vi "XYZStage-Initialisation (ver 2).vi"(8 "Error In":errorcluster, 10 "Stage Comms":T1={"CommsProtocol.lvclass"=refnum, "CommsProtocol.lvclass 2"=refnum, "CommsProtocol.lvclass 3"=refnum, "XYZ Control Config"=enum."XYZ", "Translation Stage Description"=""}, 11 "XYZ Stage Control.lvclass":refnum<class "XYZ Stage Control.lvclass">) -> (0 "Error Out":errorcluster, 3 "XYZ Stage Control out":refnum<class "XYZ Stage Control.lvclass">)   [LabVIEW 2020]
uses:
  Typedefs/Comms settings-rs232.ctl
  XYZ Stage Control/XYZ Stage Control.lvclass
  typedefs/TranslationStageControlInfo.ctl
  Generic Comms/CommsProtocol/CommsProtocol.lvclass
  typedefs/XYZControlConfig.ctl
  Globals/gl_XYZStage globals.vi
  <instrlib>/Olympus IX BX Series/Olympus IX BX Series.lvlib
  <vilib>/Instr/_visa.llb/VISA Configure Serial Port (Instr).vi
panel:
  in  "Connection Z":T3={"baud rate"=9600, "data bits"=8, "parity"=0, "stop bits"=10, "flow control"=0} {"flow control" items=["None"=0, "XON/XOFF"=1, "RTS/CTS"=2, "DTR/DSR"=4]; "stop bits" items=["1.0"=10, "1.5"=15, "2.0"=20]; "parity" items=["None", "Odd", "Even", "Mark", "Space"]; "data bits" min=5 max=8 step=1}
  out "VISA resource name out Z":refnum<visa-resource-name>
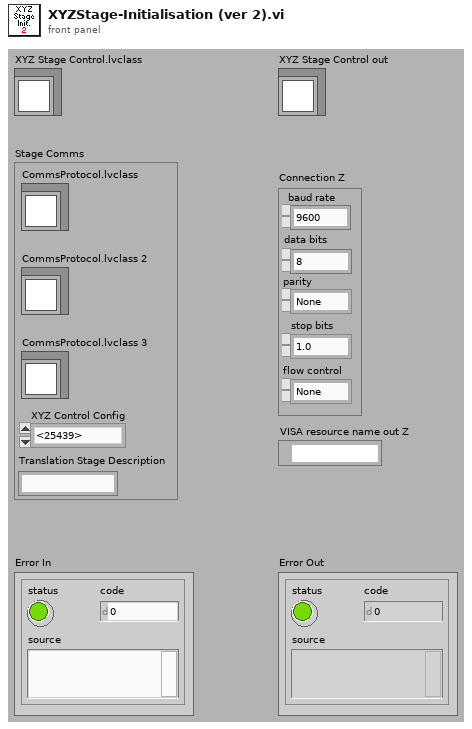
[diagram p1: front panel]
types:
  T1 = typedef "TranslationStageControlInfo.ctl" = cluster{"CommsProtocol.lvclass":refnum<class "CommsProtocol.lvclass">, "CommsProtocol.lvclass 2":refnum<class "CommsProtocol.lvclass">, "CommsProtocol.lvclass 3":refnum<class "CommsProtocol.lvclass">, "XYZ Control Config":T2, "Translation Stage Description":string}
  T2 = typedef "XYZControlConfig.ctl" = enum16{"None", "XYZ", "XY-Z", "X-Y-Z", "Z"}
  T3 = typedef "Comms settings-rs232.ctl" = cluster{"baud rate":u32, "data bits":u16, "parity":u16, "stop bits":u16, "flow control":u16}
  T4 = cluster{"Baud Rate (19200)":u32, "Flow Control (2: RTS/CTS)":u16, "Parity (2: Even)":u16, "Data Bits (8)":u16, "Stop Bits (20: 2.0)":u16}
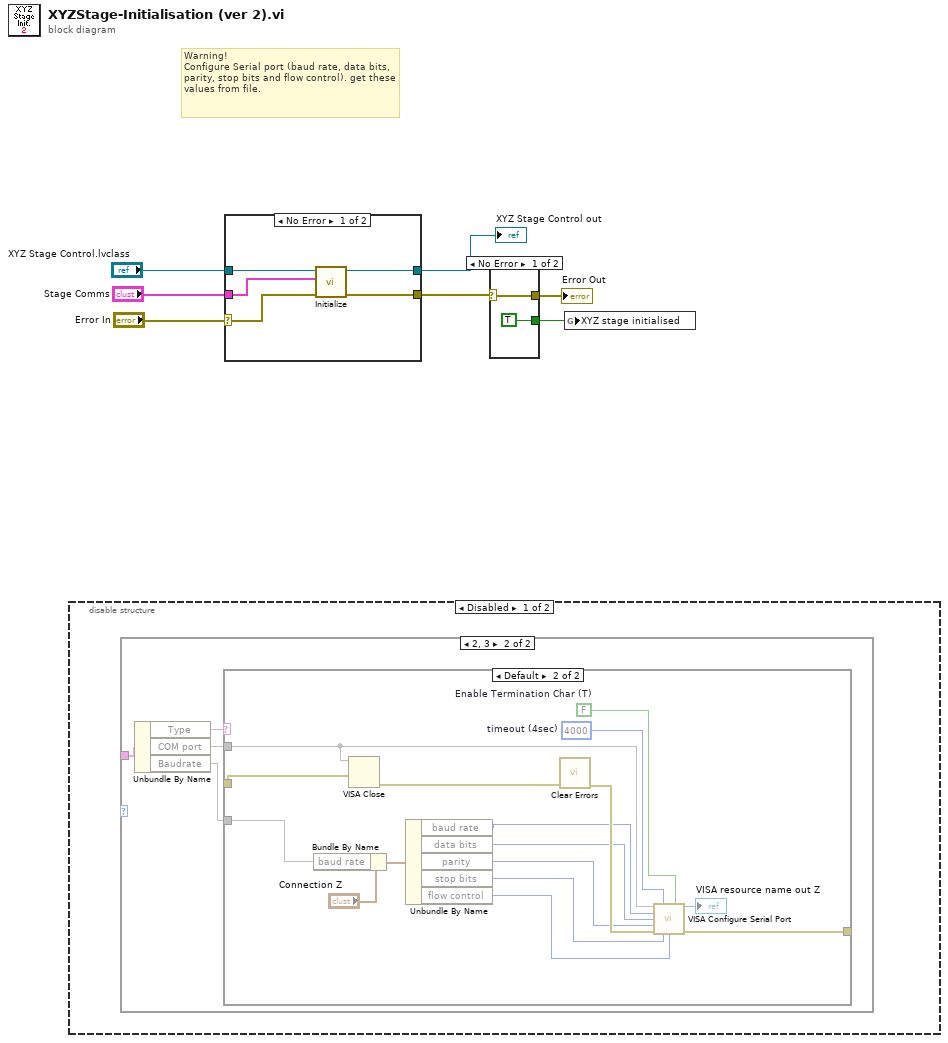
[diagram p0: block diagram]
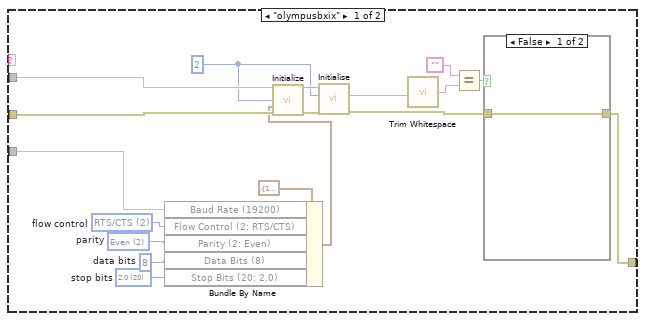
[diagram p3: hidden frame]
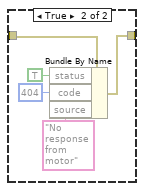
[diagram p4: hidden frame]
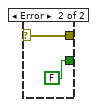
[diagram p6: hidden frame]
diagram:
  # "Warning!\nConfigure Serial port (baud rate, data bits, parity, stop bits and flow control). get these values from file."
  n1 = disable-structure shown="Disabled" {
    frame Disabled {
      n2 = case shown="2, 3" {
        selector: _ -> [_ _]
        tunnel: _ -> [_ w10]
        frame 0, Default {
        }
        frame 2, 3 {
          n3 = Unbundle By Name(w10) -> ("Type"=w8, "COM port"=w12, "Baudrate"=w11)
          n4 = case shown="Default" w8 {
            tunnel: w12 -> [w25 w49]
            tunnel: w11 -> [w26 w45]
            tunnel: [w28 w40] -> w9
            tunnel: [w20 w39] -> _
            frame "olympusbxix" {
              w18 = u16 8  # data bits
              w17 = u16 2 items=["None", "Odd", "Even", "Mark", "Space"]  # parity
              w16 = u16 20 items=["1.0"=10, "1.5"=15, "2.0"=20]  # stop bits
              w15 = u16 2 items=["None"=0, "XON/XOFF"=1, "RTS/CTS"=2, "DTR/DSR"=4]  # flow control
              w19 = 2 ("Device Number (1)")
              n5 = Bundle By Name(cluster=T4 {"Baud Rate (19200)"=19200, "Flow Control (2: RTS/CTS)"=2, "Parity (2: Even)"=2, "Data Bits (8)"=8, "Stop Bits (20: 2.0)"=20} ("Serial Configuration"), "Baud Rate (19200)"=w26, "Flow Control (2: RTS/CTS)"=w15, "Parity (2: Even)"=w17, "Data Bits (8)"=w18, "Stop Bits (20: 2.0)"=w16) -> (w24:T4)
              n6 = call <instrlib>:"Initialize.vi"("VISA Resource Name"=w25, "Device Number (1)"=w19, "Serial Configuration"=w24, "error in (no error)"=w28) -> ("VISA Resource Name Out"=w30:refnum<visa-resource-name>, "error out"=w29:errorcluster)  [unwired: 10 in]
              n7 = call "Initialise.vi"("error in (no error)"=w29, "Device Number (1)"=w19, "VISA Resource Name"=w30) -> ("error out"=w14:errorcluster, "Result"=w13:string)  [unwired: 6 in, 1 out]
              n8 = call <vilib>:"Trim Whitespace.vi"("string"=w13) -> ("trimmed string"=w23:string)  [unwired: 1 in]
              n9 = Equal?(x="", y=w23) -> (x = y?=w21:bool)
              n10 = case shown="False" w21 {
                tunnel: w14 -> [w31 w36]
                tunnel: [w31 w35] -> w20
                frame False {
                }
                frame True {
                  n11 = Bundle By Name(cluster=w36, "status"=TRUE, "code"=404, "source"="No response from motor") -> (w35:errorcluster)
                }
              }
            }
            frame Default {
              w50 = FALSE  # Enable Termination Char (T)
              w51 = u32 4000  # timeout (4sec)
              n12 = Bundle By Name(cluster="Connection Z", "baud rate"=w45) -> (w44:T3)
              n13 = VISA Close(VISA resource name=w49, error in (no error)=w40) -> (error out=w48:errorcluster)
              n14 = Unbundle By Name(w44) -> ("baud rate"=w43:u32, "data bits"=w42:u16, "parity"=w41:u16, "stop bits"=w38:u16, "flow control"=w37:u16)
              n15 = call <vilib>:"Clear Errors.vi"("error in (no error)"=w48) -> ("error out"=w47:errorcluster)  [unwired: 5 in, 1 out]
              n16 = call-poly "VISA Configure Serial Port"("VISA resource name"=w49, "timeout (10sec)"=w51, "Enable Termination\nChar (T)"=w50, "baud rate (9600)"=w43, "data bits (8)"=w42, "parity (0:none)"=w41, "error in (no error)"=w47, "stop bits (10: 1 bit)"=w38, "flow control (0:none)"=w37) -> ("VISA resource name out"=→"VISA resource name out Z":refnum<visa-resource-name>, "error out"=w39:errorcluster)  [unwired: 5 out]
            }
          }
        }
      }
    }
    frame Enabled {
    }
  }
  n17 = case shown="No Error" "Error In" {
    selector: "Error In" -> [w57 w59]
    tunnel: [w53 w59] -> w6
    tunnel: "XYZ Stage Control.lvclass" -> [w56 w58]
    tunnel: [w55 w58] -> w4
    tunnel: "Stage Comms" -> [w54 _]
    frame No Error {
      n18 = call-dynamic <instrlib>:"Initialize.vi"("error in (no error)"=w57, "Stage Comms"=w54, "XYZ Stage Control in"=w56) -> ("error out"=w53:errorcluster, "XYZ Stage Control out"=w55:refnum<class "XYZ Stage Control.lvclass">)  [unwired: 7 in]
    }
    frame Error {
    }
  }
  "XYZ Stage Control out" <- w4
  n19 = case shown="No Error" w6 {
    selector: w6 -> [w61 w62]
    tunnel: [TRUE ("XYZ stage initialised") FALSE ("XYZ stage initialised")] -> w3
    tunnel: [w61 w62] -> w5
    frame No Error {
    }
    frame Error {
    }
  }
  "Error Out" <- w5
  n20 = global write "gl_XYZStage globals.vi" "XYZ stage initialised"(w3) -> ()
